vi "Begin.vi"(8 "error in":errorcluster) -> (0 "error out":errorcluster)   [LabVIEW 2020]
doc: "Called before other user functions, this VI is expected to open initial I/O refnums, load in file data, and do all program initialization. Notice that the <B>error out</B> terminal is simply used for data flow. Wiring it to other structures or subVIs ensures that this VI runs first."
uses:
  <vilib>/Rock Robotics/WPI/DriverStation/WPI_DriverStationRobotMode2.ctl
  <vilib>/Rock Robotics/WPI/Joystick/WPI_JoystickDeviceEnum.ctl
  <vilib>/Rock Robotics/WPI/RobotDrive/WPI_RobotDriveDevRef.ctl
  <vilib>/Rock Robotics/WPI/MotorControl/WPI_MotorControlDeviceRef.ctl
  <vilib>/Rock Robotics/WPI/MotorControl/WPI_MotorControlType.ctl
  <vilib>/Rock Robotics/SystemInterfaces/DIO/FPGA_DIOPWMChannel.ctl
  <vilib>/Rock Robotics/WPI/PWM/WPI_PWMDeadband.ctl
  <vilib>/Rock Robotics/SystemInterfaces/DIO/FPGA_DIOChannel.ctl
  <vilib>/Rock Robotics/WPI/SafetyOutput/WPI_SafetyOutputConfigMenu.ctl
  <vilib>/Rock Robotics/WPI/Solenoid/WPI_SolenoidChannel.ctl
  <vilib>/Rock Robotics/WPI/ThirdParty/REV Robotics/REVLib/Typedef/Spark MAX Idle Mode.ctl
  <vilib>/Rock Robotics/WPI/ThirdParty/REV Robotics/REVLib/Typedef/Spark MAX Motor Type.ctl
  Robot Global Data.vi
  <vilib>/Rock Robotics/Network Tables/NT Write String Array.vi
  <vilib>/Rock Robotics/WPI/Utilities/WPI_GetSetVariantRefNum.vi
  <vilib>/Rock Robotics/WPI/Solenoid/WPI_SolenoidOpenSingle.vi
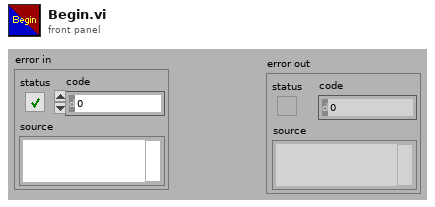
[diagram p1: front panel]
types:
  T1 = typedef "WPI_JoystickDeviceEnum.ctl" = enum16{"USB 0", "USB 1", "USB 2", "USB 3", "USB 4", "USB 5"}
  T2 = typedef "FPGA_DIOChannel.ctl" = enum8{"DIO 0", "DIO 1", "DIO 2", "DIO 3", "DIO 4", "DIO 5", "DIO 6", "DIO 7", "DIO 8", "DIO 9", "DIO MXP 0", "DIO MXP 1", "DIO MXP 2", "DIO MXP 3", "DIO MXP 4", "DIO MXP 5", "DIO MXP 6", "DIO MXP 7", "DIO MXP 8", "DIO MXP 9", "DIO MXP 10", "DIO MXP 11", "DIO MXP 12", "DIO MXP 13", "DIO MXP 14", "DIO MXP 15", "SPI Port CS1", "SPI Port CS2", "SPI Port CS3", "SPI Port MISO", "SPI Port MOSI", "Invalid"}
  T3 = typedef "WPI_SafetyOutputConfigMenu.ctl" = enum16{"Enable", "Disable"}
  T4 = typedef "WPI_SolenoidChannel.ctl" = enum8{"Solenoid 0", "Solenoid 1", "Solenoid 2", "Solenoid 3", "Solenoid 4", "Solenoid 5", "Solenoid 6", "Solenoid 7", "Solenoid 8", "Solenoid 9", "Solenoid 10", "Solenoid 11", "Solenoid 12", "Solenoid 13", "Solenoid 14", "Solenoid 15", "Invalid"}
  T5 = typedef "WPI_RobotDriveDevRef.ctl" = cluster{"DevStatus":errorcluster, "Motors[]":T6[], "Square Inputs":bool, "Max Output":dbl}
  T6 = typedef "WPI_MotorControlDeviceRef.ctl" = cluster{"DeviceStatus":errorcluster, "Type":T7, "PWM":cluster{"PWM Channel":T8, "DeadBand":T9}, "CAN":cluster{"Device Number":u8, "SetOutput VI Ref":variant, "GetOutput VI Ref":variant, "Enable VI Ref":variant, "Disable VI Ref":variant, "Data":variant}, "Invert":bool, "DIO PWM":cluster{"PWM \"Enable\" Channel":T8, "DIOChannel":T2, "PWM Rate":dbl}}
  T7 = typedef "WPI_MotorControlType.ctl" = enum16{"PWM", "CAN", "DIO PWM"}
  T8 = typedef "FPGA_DIOPWMChannel.ctl" = enum8{"PWM 0", "PWM 1", "PWM 2", "PWM 3", "PWM 4", "PWM 5", "PWM 6", "PWM 7", "PWM 8", "PWM 9", "PWM MXP 0", "PWM MXP 1", "PWM MXP 2", "PWM MXP 3", "PWM MXP 4", "PWM MXP 5", "PWM MXP 6", "PWM MXP 7", "PWM MXP 8", "PWM MXP 9", "Invalid"}
  T9 = typedef "WPI_PWMDeadband.ctl" = cluster{"Name":string, "maxPositivePwm":i32, "minPositivePwm":i32, "centerPwm":i32, "maxNegativePwm":i32, "minNegativePwm":i32, "angularRange":u16}
  T10 = typedef "WPI_DriverStationRobotMode2.ctl" = enum16{"Autonomous Disabled", "Autonomous Enabled", "Teleop Disabled", "Teleop Enabled", "Disconnected", "Finish", "Test Disabled", "Test Enabled", "Emergency Stopped"}
  T11 = typedef "WPI_SolenoidDevRef.ctl" = cluster{"DevStatus":errorcluster, "Pneumatics Control Module":u8, "Forward Solenoid Channel":T4, "Reverse Solenoid Channel":T4}
  T12 = typedef "WPI_CompressorDevRef.ctl" = cluster{"DevStatus":errorcluster, "Pneumatics Control Module":u8}
  T13 = typedef "WPI_JoystickDevRef.ctl" = cluster{"Device":T1}
  T14 = typedef "Spark MAX Motor Type.ctl" = enum16{"Brushed", "Brushless"}
  T15 = typedef "Spark MAX Idle Mode.ctl" = enum16{"Coast", "Brake"}
  T16 = typedef "WPI_DigitalInputDevRef.ctl" = cluster{"DevStatus":errorcluster, "DIO Channel":T2}
  T17 = cluster{"Motors[][0]":T6, "Motors[][1]":T6, "Motors[][2]":T6, "Motors[][3]":T6, "Motors[][4]":T6, "Motors[][5]":T6, "Motors[][6]":T6, "Motors[][7]":T6, "Motors[][8]":T6}
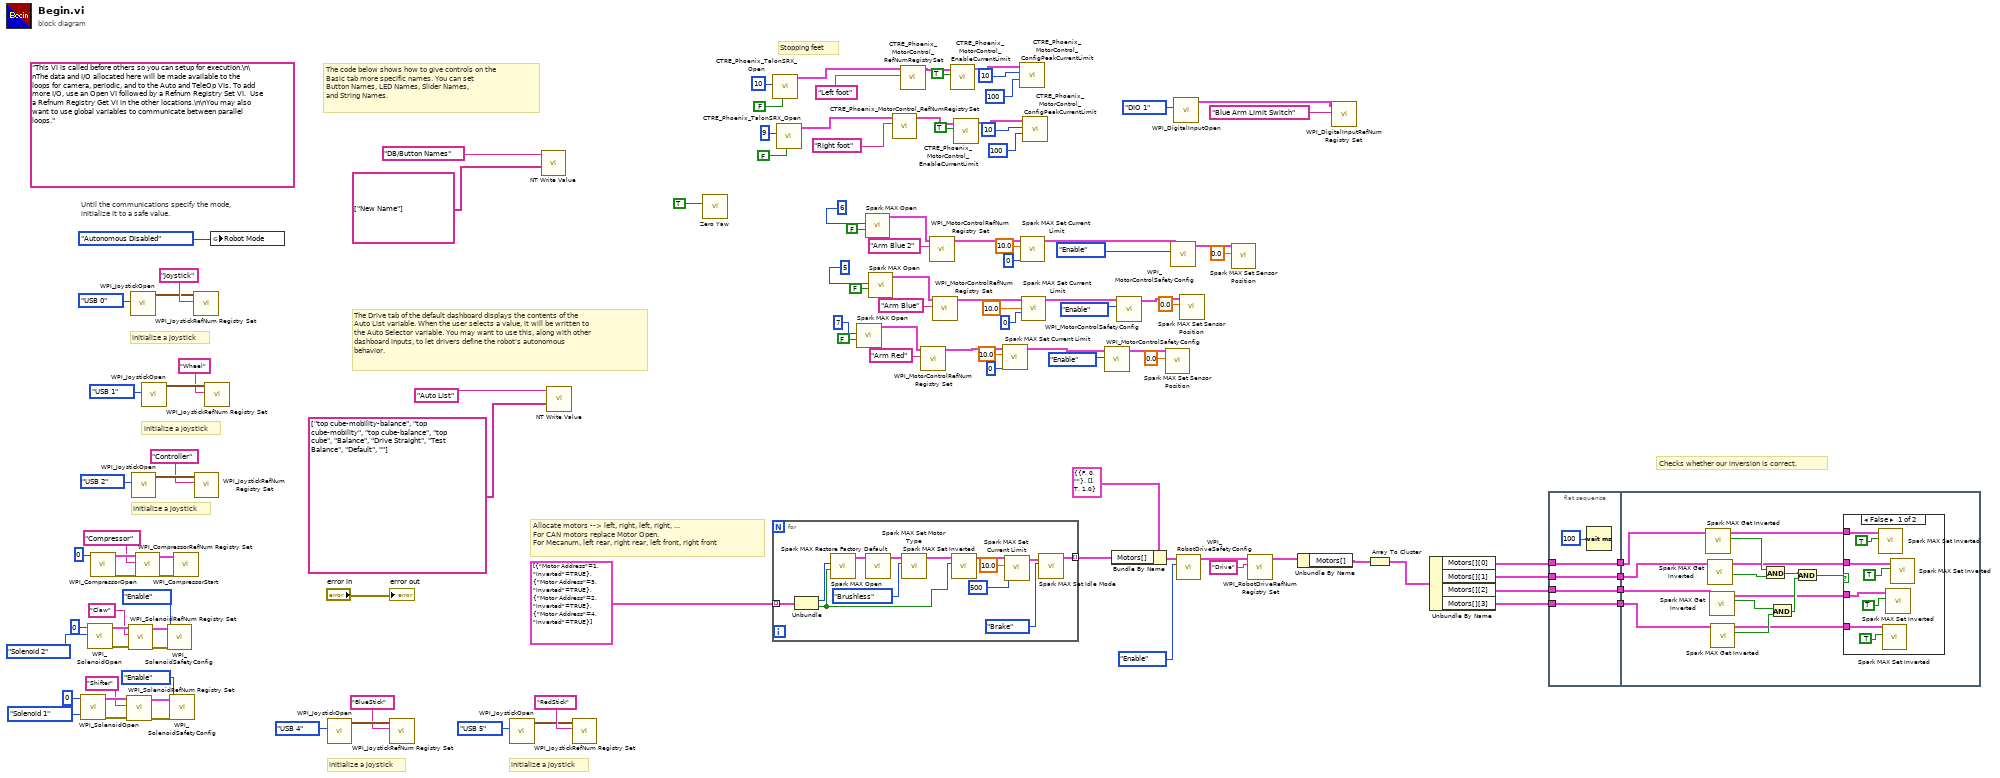
[diagram p0: block diagram]
diagram:
  (unwired) "This VI is called before others so you can setup for execution.\n\nThe data and I/O allocated here will be made available to the loops for camera, periodic, and to the Auto and TeleOp VIs. To add more I/O, use an Open VI followed by a Refnum Registry Set VI.  Use a Refnum Registry Get VI in the other locations.\n\nYou may also want to use global variables to communicate between parallel loops."
  # "initialize a joystick"
  # "initialize a joystick"
  # "Stopping feet"
  # "Checks whether our inversion is correct."
  # "initialize a joystick"
  # "initialize a joystick"
  # "Allocate motors --> left, right, left, right, ... \nFor CAN motors replace Motor Open.\nFor Mecanum, left rear, right rear, left front, right front"
  # "The Drive tab of the default dashboard displays the contents of the\nAuto List variable. When the user selects a value, it will be written to\nthe Auto Selector variable. You may want to use this, along with other\ndashboard inputs, to let drivers define the robot's autonomous\nbehavior."
  # "The code below shows how to give controls on the\nBasic tab more specific names. You can set\nButton Names, LED Names, Slider Names,\nand String Names."
  # "initialize a joystick"
  # "Until the communications specify the mode,\ninitialize it to a safe value."
  n1 = call-poly <vilib>:"WPI_SolenoidOpen.vi"("Solenoid Channel"=WPI_SolenoidChannel."Solenoid 1", "Pneumatics Device (def)"=u8 0) -> ("error out"=w75:errorcluster, "SolenoidDevRef"=w74:T11)  [unwired: 8 in]
  n2 = call-poly <vilib>:"WPI_SolenoidOpen.vi"("Solenoid Channel"=WPI_SolenoidChannel."Solenoid 2", "Pneumatics Device (def)"=u8 0) -> ("error out"=w77:errorcluster, "SolenoidDevRef"=w76:T11)  [unwired: 8 in]
  n3 = call <vilib>:"WPI_CompressorOpen.vi"("Pneumatics device (def)"=u8 0) -> ("CompressorDevRef"=w82:T12, "error out"=w83:errorcluster)  [unwired: 13 in]
  n4 = call <vilib>:"WPI_SolenoidRefNum Registry Set.vi"("error in (no error)"=w75, "refnum name"="Shifter", "SolenoidDevRef"=w74) -> ("error out"=w66:errorcluster, "SolenoidDevRef"=w65:T11)  [unwired: 7 in]
  n5 = call <vilib>:"WPI_SolenoidRefNum Registry Set.vi"("error in (no error)"=w77, "refnum name"="Claw", "SolenoidDevRef"=w76) -> ("error out"=w69:errorcluster, "SolenoidDevRef"=w68:T11)  [unwired: 7 in]
  n6 = call <vilib>:"WPI_JoystickOpen.vi"("JoystickDevice"=WPI_JoystickDeviceEnum."USB 0") -> ("JoystickDevRef"=w114:T13)  [unwired: 10 in]
  n7 = call <vilib>:"WPI_JoystickOpen.vi"("JoystickDevice"=WPI_JoystickDeviceEnum."USB 2") -> ("JoystickDevRef"=w97:T13)  [unwired: 10 in]
  n8 = call <vilib>:"WPI_CompressorRefNum Registry Set.vi"("error in (no error)"=w83, "refnum name"="Compressor", "CompressorDevRef"=w82) -> ("error out"=w79:errorcluster, "CompressorDevRef"=w78:T12)  [unwired: 7 in]
  n9 = call <vilib>:"WPI_JoystickOpen.vi"("JoystickDevice"=WPI_JoystickDeviceEnum."USB 1") -> ("JoystickDevRef"=w100:T13)  [unwired: 10 in]
  n10 = call <vilib>:"WPI_SolenoidSafetyConfig.vi"("error in (no error)"=w69, "mode"=WPI_SafetyOutputConfigMenu."Enable", "SolenoidDevRef"=w68) -> ()  [unwired: 7 in, 2 out]
  n11 = call <vilib>:"WPI_SolenoidSafetyConfig.vi"("error in (no error)"=w66, "mode"=WPI_SafetyOutputConfigMenu."Enable", "SolenoidDevRef"=w65) -> ()  [unwired: 7 in, 2 out]
  n12 = call <vilib>:"WPI_CompressorStart.vi"("error in (no error)"=w79, "CompressorDevRef"=w78) -> ()  [unwired: 8 in, 2 out]
  n13 = call <vilib>:"WPI_JoystickRefNum Registry Set.vi"("refnum name"="Joystick", "JoystickDevRef"=w114) -> ()  [unwired: 8 in, 2 out]
  n14 = call <vilib>:"WPI_JoystickRefNum Registry Set.vi"("refnum name"="Controller", "JoystickDevRef"=w97) -> ()  [unwired: 8 in, 2 out]
  n15 = call <vilib>:"WPI_JoystickRefNum Registry Set.vi"("refnum name"="Wheel", "JoystickDevRef"=w100) -> ()  [unwired: 8 in, 2 out]
  n16 = global write "Robot Global Data.vi" "Robot Mode"(WPI_DriverStationRobotMode2."Autonomous Disabled" ("Robot Mode")) -> ()
  n17 = call <vilib>:"WPI_JoystickOpen.vi"("JoystickDevice"=WPI_JoystickDeviceEnum."USB 4") -> ("JoystickDevRef"=w5:T13)  [unwired: 10 in]
  n18 = call <vilib>:"WPI_JoystickRefNum Registry Set.vi"("refnum name"="BlueStick", "JoystickDevRef"=w5) -> ()  [unwired: 8 in, 2 out]
  n19 = call <vilib>:"WPI_JoystickOpen.vi"("JoystickDevice"=WPI_JoystickDeviceEnum."USB 5") -> ("JoystickDevRef"=w2:T13)  [unwired: 10 in]
  n20 = call-poly <vilib>:"NT Write Value.vi"("value"=string[] ["New Name"], "name"="DB/Button Names" ("Name")) -> ()  [unwired: 9 in, 1 out]
  n21 = call-poly <vilib>:"NT Write Value.vi"("value"=string[] ["top cube-mobility-balance", "top cube-mobility", "top cube-balance", "top cube", "Balance", "Drive Straight", "Test Balance", "Default", ""] ("String Array"), "name"="Auto List" ("Name")) -> ()  [unwired: 9 in, 1 out]
  n22 = call <vilib>:"WPI_JoystickRefNum Registry Set.vi"("refnum name"="RedStick", "JoystickDevRef"=w2) -> ()  [unwired: 8 in, 2 out]
  n23 = call <vilib>:"Zero Yaw.vi"("Zero"=TRUE) -> ()  [unwired: 11 in]
  n24 = call <vilib>:"CTRE_Phoenix_TalonSRX_Open.vi"("Invert"=FALSE, "Device Number"=u8 10) -> ("PhoenixMotorControlDevRef"=w45:T6)  [unwired: 8 in, 1 out]
  n25 = for {
    tunnel: cluster{"Motor Address":i32, "Inverted":bool}[] [{"Motor Address"=1, "Inverted"=TRUE}, {"Motor Address"=3, "Inverted"=TRUE}, {"Motor Address"=2, "Inverted"=TRUE}, {"Motor Address"=4, "Inverted"=TRUE}] ("Array") -> [w129] mode=indexing
    tunnel: [w126] -> w84 mode=indexing
    n26 = Unbundle(w129) -> ("Motor Address"=w128:i32, "Inverted"=w122:bool)
    n27 = call <vilib>:"Spark MAX Open.vi"("Invert"=w122, "Device Number"=w128) -> ("MotorControlDeviceRef"=w125:T6)  [unwired: 8 in, 1 out]
    n28 = call <vilib>:"Spark MAX Restore Factory Default.vi"("MotorControlDeviceRef"=w125) -> ("MotorControlDeviceRef"=w124:T6)  [unwired: 9 in, 1 out]
    n29 = call <vilib>:"Spark MAX Set Motor Type.vi"("Motor Type"=Spark_MAX_Motor_Type."Brushless", "MotorControlDevRef"=w124) -> ("MotorControlDeviceRef"=w123:T6)  [unwired: 8 in, 1 out]
    n30 = call <vilib>:"Spark MAX Set Inverted.vi"("Inverted (F)"=w122, "MotorControlDeviceRef in"=w123) -> ("MotorControlDeviceRef out"=w119:T6)  [unwired: 8 in, 1 out]
    n31 = call <vilib>:"Spark MAX Set Current Limit.vi"("Limit Duration (0)"=u32 500, "Current Limit A (100)"=sgl 10.0, "MotorControlDeviceRef in"=w119) -> ("MotorControlDeviceRef out"=w120:T6)  [unwired: 7 in, 1 out]
    n32 = call <vilib>:"Spark MAX Set Idle Mode.vi"("Idle Mode"=Spark_MAX_Idle_Mode."Brake", "MotorControlDeviceRef in"=w120) -> ("MotorControlDeviceRef out"=w126:T6)  [unwired: 8 in, 1 out]
  }
  n33 = call <vilib>:"CTRE_Phoenix_TalonSRX_Open.vi"("Invert"=FALSE, "Device Number"=u8 9) -> ("PhoenixMotorControlDevRef"=w42:T6)  [unwired: 8 in, 1 out]
  n34 = call <vilib>:"Spark MAX Open.vi"("Invert"=FALSE, "Device Number"=u8 7) -> ("MotorControlDeviceRef"=w94:T6)  [unwired: 8 in, 1 out]
  n35 = call <vilib>:"Spark MAX Open.vi"("Invert"=FALSE, "Device Number"=u8 6) -> ("MotorControlDeviceRef"=w59:T6)  [unwired: 8 in, 1 out]
  n36 = call <vilib>:"Spark MAX Open.vi"("Invert"=FALSE, "Device Number"=u8 5) -> ("MotorControlDeviceRef"=w89:T6)  [unwired: 8 in, 1 out]
  n37 = call <vilib>:"CTRE_Phoenix_MotorControl_RefNumRegistrySet.vi"("refnum name"="Right foot", "PhoenixMotorControlDevRef"=w42) -> ("PhoenixMotorControlDevRef"=w16:T6)  [unwired: 8 in, 1 out]
  n38 = call <vilib>:"CTRE_Phoenix_MotorControl_RefNumRegistrySet.vi"("refnum name"="Left foot", "PhoenixMotorControlDevRef"=w45) -> ("PhoenixMotorControlDevRef"=w25:T6)  [unwired: 8 in, 1 out]
  n39 = call <vilib>:"WPI_MotorControlRefNum Registry Set.vi"("refnum name"="Arm Red", "MotorControlDevRef"=w94) -> ("MotorControlDevRef"=w33:T6)  [unwired: 8 in, 1 out]
  n40 = call <vilib>:"WPI_MotorControlRefNum Registry Set.vi"("refnum name"="Arm Blue 2", "MotorControlDevRef"=w59) -> ("MotorControlDevRef"=w37:T6)  [unwired: 8 in, 1 out]
  n41 = call <vilib>:"WPI_MotorControlRefNum Registry Set.vi"("refnum name"="Arm Blue", "MotorControlDevRef"=w89) -> ("MotorControlDevRef"=w35:T6)  [unwired: 8 in, 1 out]
  n42 = call <vilib>:"CTRE_Phoenix_MotorControl_EnableCurrentLimit.vi"("Enable Current Limit?"=TRUE, "PhoenixMotorControlDevRef"=w25) -> ("PhoenixMotorControlDevRef"=w24:T6)  [unwired: 8 in, 1 out]
  n43 = call <vilib>:"CTRE_Phoenix_MotorControl_EnableCurrentLimit.vi"("Enable Current Limit?"=TRUE, "PhoenixMotorControlDevRef"=w16) -> ("PhoenixMotorControlDevRef"=w17:T6)  [unwired: 8 in, 1 out]
  n44 = call <vilib>:"Spark MAX Set Current Limit.vi"("Limit Duration (0)"=u32 0, "Current Limit A (100)"=sgl 10.0, "MotorControlDeviceRef in"=w33) -> ("MotorControlDeviceRef out"=w32:T6)  [unwired: 7 in, 1 out]
  n45 = call <vilib>:"CTRE_Phoenix_MotorControl_ConfigPeakCurrentLimit.vi"("Peak Current Maximum Duration (ms)"=100, "Peak Current (Amps)"=10, "PhoenixMotorControlDevRef"=w24) -> ()  [unwired: 7 in, 2 out]
  n46 = call <vilib>:"Spark MAX Set Current Limit.vi"("Limit Duration (0)"=u32 0, "Current Limit A (100)"=sgl 10.0, "MotorControlDeviceRef in"=w37) -> ("MotorControlDeviceRef out"=w36:T6)  [unwired: 7 in, 1 out]
  n47 = call <vilib>:"Spark MAX Set Current Limit.vi"("Limit Duration (0)"=u32 0, "Current Limit A (100)"=sgl 10.0, "MotorControlDeviceRef in"=w35) -> ("MotorControlDeviceRef out"=w34:T6)  [unwired: 7 in, 1 out]
  n48 = call <vilib>:"CTRE_Phoenix_MotorControl_ConfigPeakCurrentLimit.vi"("Peak Current Maximum Duration (ms)"=100, "Peak Current (Amps)"=10, "PhoenixMotorControlDevRef"=w17) -> ()  [unwired: 7 in, 2 out]
  n49 = call <vilib>:"WPI_MotorControlSafetyConfig.vi"("mode"=WPI_SafetyOutputConfigMenu."Enable", "MotorControlDevRef"=w32) -> ("MotorControlDevRef"=w10:T6)  [unwired: 8 in, 1 out]
  n50 = Bundle By Name(cluster=T5 {"DevStatus"={"status"=FALSE, "code"=0, "source"=""}, "Motors[]"=[], "Square Inputs"=TRUE, "Max Output"=1.0} ("RobotDriveDevRef"), "Motors[]"=w84) -> (w106:T5)
  n51 = call <vilib>:"WPI_MotorControlSafetyConfig.vi"("mode"=WPI_SafetyOutputConfigMenu."Enable", "MotorControlDevRef"=w34) -> ("MotorControlDevRef"=w15:T6)  [unwired: 8 in, 1 out]
  n52 = call <vilib>:"Spark MAX Set Sensor Position.vi"("Position"=0.0, "MotorControlDeviceRef"=w10) -> ()  [unwired: 8 in, 2 out]
  n53 = call <vilib>:"WPI_MotorControlSafetyConfig.vi"("mode"=WPI_SafetyOutputConfigMenu."Enable", "MotorControlDevRef"=w36) -> ("MotorControlDevRef"=w11:T6)  [unwired: 8 in, 1 out]
  n54 = call <vilib>:"WPI_DigitalInputOpen.vi"("DIO Channel"=FPGA_DIOChannel."DIO 1") -> ("DigitalInputDevRef"=w7:T16)  [unwired: 9 in, 1 out]
  n55 = call <vilib>:"WPI_RobotDriveSafetyConfig.vi"("mode"=WPI_SafetyOutputConfigMenu."Enable", "RobotDriveDevRef"=w106) -> ("RobotDriveDevRef"=w103:T5)  [unwired: 2 in, 7 out]
  n56 = call <vilib>:"Spark MAX Set Sensor Position.vi"("Position"=0.0, "MotorControlDeviceRef"=w15) -> ()  [unwired: 8 in, 2 out]
  n57 = call <vilib>:"Spark MAX Set Sensor Position.vi"("Position"=0.0, "MotorControlDeviceRef"=w11) -> ()  [unwired: 8 in, 2 out]
  n58 = call <vilib>:"WPI_RobotDriveRefNum Registry Set.vi"("refnum name"="Drive", "RobotDriveDevRef"=w103) -> ("RobotDriveDevRef"=w54:T5)  [unwired: 8 in, 1 out]
  n59 = Unbundle By Name(w54) -> ("Motors[]"=w56:T6[])
  n60 = call <vilib>:"WPI_DigitalInputRefNum Registry Set.vi"("refnum name"="Blue Arm Limit Switch", "DigitalInputDevRef"=w7) -> ()  [unwired: 8 in, 2 out]
  n61 = Array To Cluster(array=w56) -> (cluster=w55:T17)
  n62 = Unbundle By Name(w55) -> ("Motors[][0]"=w52:T6, "Motors[][1]"=w50:T6, "Motors[][2]"=w48:T6, "Motors[][3]"=w46:T6)
  n63 = flat-sequence {
    tunnel: [w133] -> w53
    tunnel: w52 -> [w133]
    tunnel: [w132] -> w51
    tunnel: w50 -> [w132]
    tunnel: [w131] -> w49
    tunnel: w48 -> [w131]
    tunnel: [w130] -> w47
    tunnel: w46 -> [w130]
    tunnel: w53 -> [w138]
    tunnel: w51 -> [w137]
    tunnel: w49 -> [w136]
    tunnel: w47 -> [w135]
    frame #0 {
      n64 = Wait (ms)(milliseconds to wait=u32 100) -> ()  [unwired: 1 out]
    }
    frame #1 {
      n65 = call <vilib>:"Spark MAX Get Inverted.vi"("MotorControlDeviceRef in"=w138) -> ("Inverted"=w149:bool, "MotorControlDeviceRef out"=w142:T6)  [unwired: 8 in, 1 out]
      n66 = call <vilib>:"Spark MAX Get Inverted.vi"("MotorControlDeviceRef in"=w137) -> ("Inverted"=w148:bool, "MotorControlDeviceRef out"=w141:T6)  [unwired: 8 in, 1 out]
      n67 = call <vilib>:"Spark MAX Get Inverted.vi"("MotorControlDeviceRef in"=w136) -> ("Inverted"=w147:bool, "MotorControlDeviceRef out"=w140:T6)  [unwired: 8 in, 1 out]
      n68 = call <vilib>:"Spark MAX Get Inverted.vi"("MotorControlDeviceRef in"=w135) -> ("Inverted"=w146:bool, "MotorControlDeviceRef out"=w139:T6)  [unwired: 8 in, 1 out]
      n69 = And(x=w149, y=w148) -> (x .and. y?=w144:bool)
      n70 = And(x=w147, y=w146) -> (x .and. y?=w145:bool)
      n71 = And(x=w144, y=w145) -> (x .and. y?=w143:bool)
      n72 = case shown="False" w143 {
        tunnel: w142 -> [w157 _]
        tunnel: w141 -> [w156 _]
        tunnel: w140 -> [w155 _]
        tunnel: w139 -> [w154 _]
        frame False {
          n73 = call <vilib>:"Spark MAX Set Inverted.vi"("Inverted (F)"=TRUE, "MotorControlDeviceRef in"=w157) -> ()  [unwired: 8 in, 2 out]
          n74 = call <vilib>:"Spark MAX Set Inverted.vi"("Inverted (F)"=TRUE, "MotorControlDeviceRef in"=w154) -> ()  [unwired: 8 in, 2 out]
          n75 = call <vilib>:"Spark MAX Set Inverted.vi"("Inverted (F)"=TRUE, "MotorControlDeviceRef in"=w155) -> ()  [unwired: 8 in, 2 out]
          n76 = call <vilib>:"Spark MAX Set Inverted.vi"("Inverted (F)"=TRUE, "MotorControlDeviceRef in"=w156) -> ()  [unwired: 8 in, 2 out]
        }
        frame True {
        }
      }
    }
  }
  "error out" <- "error in"
